vi "Key - Cluster Write.vi"(8 "error in (no error)":errorcluster, 10 "Cluster Ref in":refnum<vi>, 11 "Refnum in":T1) -> (0 "error out":errorcluster, 3 "Refnum out":T1)   [LabVIEW 2013]
uses:
  <vilib>/Utility/config.llb/Config Data RefNum.ctl
  <vilib>/Utility/config.llb/Write Key (String).vi
  <vilib>/Utility/config.llb/NI_LVConfig.lvlib
panel:
  out "Array":string[](array[string])
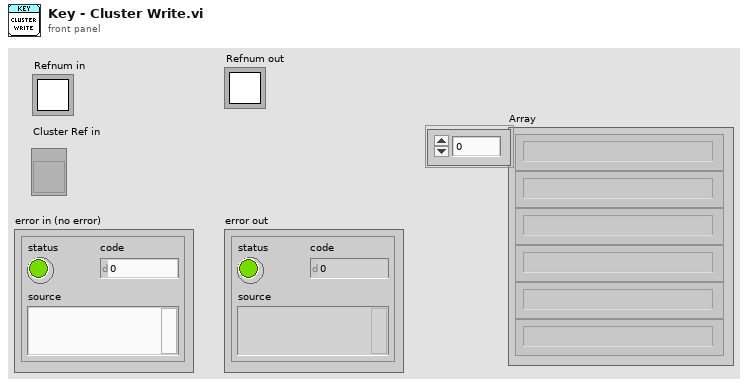
[diagram p1: front panel]
types:
  T1 = typedef "NI_LVConfig.lvlib/Config Data RefNum.ctl" = refnum<k1>
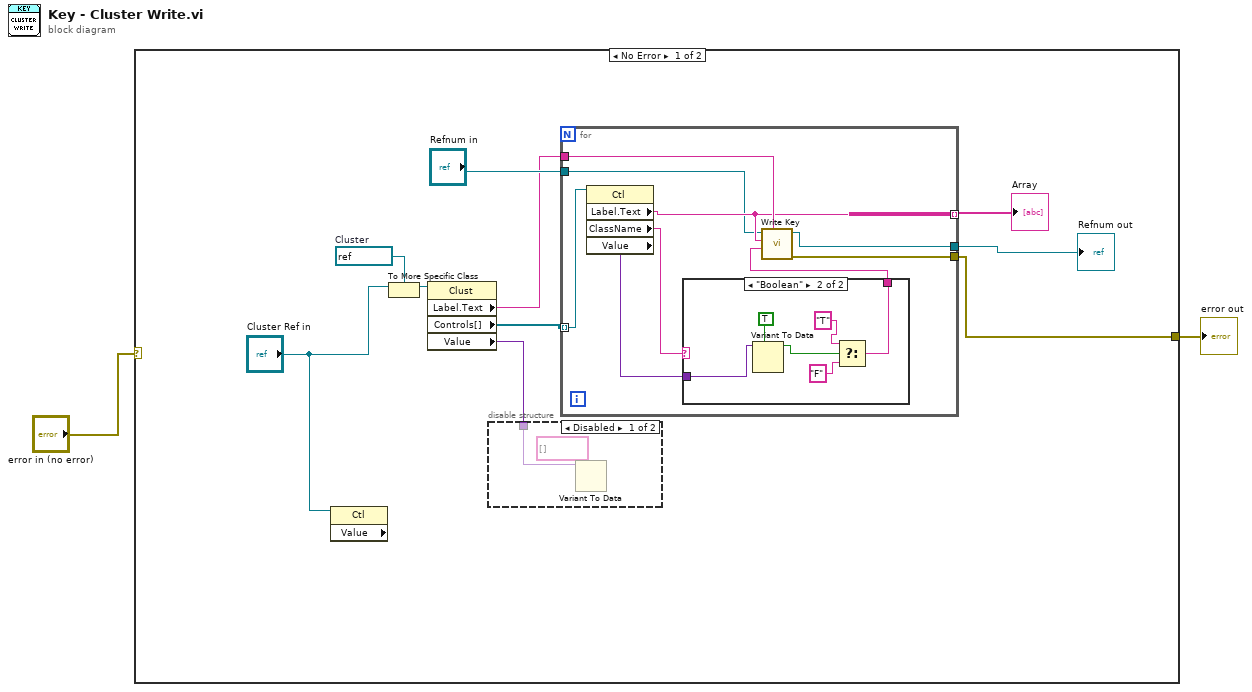
[diagram p0: block diagram]
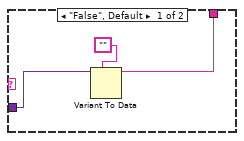
[diagram p3: hidden frame]
diagram:
  n1 = case shown="No Error" "error in (no error)" {
    selector: "error in (no error)" -> [_ w33]
    tunnel: [w5 w33] -> w2
    frame No Error {
      w12 = refnum<vi> refnum  # Cluster
      n2 = property class="Ctl" props=["Value"](reference="Cluster Ref in") -> ()  [unwired: 1 in, 3 out]
      n3 = To More Specific Class(target class=w12, reference="Cluster Ref in") -> (specific class reference=w11:refnum<vi>)  [unwired: 1 in, 1 out]
      n4 = property class="Clust"(reference=w11) -> ("Label.Text"=w7:string, "Controls[]"=w10:refnum<vi>[], "Value"=w4:variant)  [unwired: 1 in, 2 out]
      n5 = disable-structure shown="Disabled" {
        disable-tunnel: w4 -> [w13 _]
        frame Disabled {
          n6 = Variant To Data(type=string[] [], Variant=w13) -> ()  [unwired: 1 in, 2 out]
        }
        frame Enabled {
        }
      }
      n7 = for {
        tunnel: w10 -> [w23] mode=indexing
        tunnel: "Refnum in" -> [w20]
        tunnel: [w21] -> w8 mode=indexing
        tunnel: w7 -> [w22]
        tunnel: [w19] -> w6
        tunnel: [w18] -> w5
        n8 = property class="Ctl"(reference=w23) -> ("Label.Text"=w21:string, "ClassName"=w17:string, "Value"=w16:variant)  [unwired: 1 in, 2 out]
        n9 = case shown="\"Boolean\"" w17 {
          tunnel: w16 -> [w25 w32]
          tunnel: [w24 w27] -> w15
          frame "False", Default {
            n10 = Variant To Data(type="", Variant=w25) -> (data=w24:string)  [unwired: 1 in, 1 out]
          }
          frame "Boolean" {
            n11 = Variant To Data(type=TRUE, Variant=w32) -> (data=w30:bool)  [unwired: 1 in, 1 out]
            n12 = Select(t="T", s=w30, f="F") -> (s? t:f=w27:string)
          }
        }
        n13 = call-poly <vilib>:"Write Key.vi"("section"=w22, "value"=w15, "key"=w21, "refnum"=w20) -> ("error out"=w18:errorcluster, "refnum out"=w19:T1)  [unwired: 5 in, 1 out]
      }
      "Refnum out" <- w6
      "Array" <- w8
    }
    frame Error {
    }
  }
  "error out" <- w2
